vi "test_read-nmea-data2.vi"() -> ()   [LabVIEW 2019] (continued)
64,049,27,1*67\n\t\n15:12:51.40\tF9P\t$GPGSV,3,2,09,09,45,074,30,12,23,276,27,17,33,154,28,19,52,157,33,1*60\n\t\n15:12:51.42\tF9P\t$GPGSV,3,3,09,25,12,306,31,1*5E\n\t\n15:12:51.44\tF9P\t$GPGSV,3,1,09,02,55,319,,04,18,043,18,05,37,247,24,06,64,049,23,6*6C\n\t\n15:12:51.46\tF9P\t$GPGSV,3,2,09,09,45,074,27,12,23,276,,17,33,154,16,19,52,157,,6*69\n\t\n15:12:51.48\tF9P\t$GPGSV,3,3,09,25,12,306,20,6*59\n\t\n15:12:51.50\tF9P\t$GLGSV,2,1,08,69,12,031,24,70,71,039,26,71,52,205,45,72,04,209,23,1*78\n\t\n15:12:51.52\tF9P\t$GLGSV,2,2,08,77,01,326,,84,20,122,10,85,70,067,38,86,37,330,,1*72\n\t\n15:12:51.54\tF9P\t$GLGSV,2,1,08,69,12,031,17,70,71,039,,71,52,205,24,72,04,209,,3*78\n\t\n15:12:51.56\tF9P\t$GLGSV,2,2,08,77,01,326,,84,20,122,,85,70,067,21,86,37,330,,3*79\n\t\n15:12:51.58\tF9P\t$GAGSV,2,1,08,02,08,297,29,04,66,116,27,09,32,193,38,11,72,359,29,7*7B\n\t\n15:12:51.60\tF9P\t$GAGSV,2,2,08,12,40,103,33,19,26,045,19,25,09,249,,36,26,308,23,7*71\n\t\n15:12:51.62\tF9P\t$GAGSV,2,1,08,02,08,297,,04,66,116,,09,32,193,,11,72,359,,2*70\n\t\n15:12:51.64\tF9P\t$GAGSV,2,2,08,12,40,103,,19,26,045,,25,09,249,,36,26,308,,2*7D\n\t\n15:12:51.66\tF9P\t$GBGSV,1,1,04,11,49,132,31,14,87,114,28,28,,,22,33,61,220,33,1*44\n\t\n15:12:51.68\tF9P\t$GBGSV,1,1,04,10,,,33,11,49,132,,14,87,114,,33,61,220,,3*45\n\t\n15:12:51.70\tF9P\t$GNGLL,3723.54935,N,12656.96073,E,061253.00,A,A*72\n\t\n15:12:51.72\tF9P\t\t\n15:12:51.74\tF9P\t\t\n15:12:51.76\tF9P\t\t\n15:12:51.78\tF9P\t\t\n15:12:51.80\tF9P\t\t\n15:12:51.82\tF9P\t\t\n15:12:51.84\tF9P\t\t\n15:12:51.86\tF9P\t\t\n15:12:51.88\tF9P\t\t\n15:12:51.90\tF9P\t\t\n15:12:51.92\tF9P\t\t\n15:12:51.94\tF9P\t\t\n15:12:51.96\tF9P\t\t\n15:12:51.98\tF9P\t\t\n15:12:52.00\tF9P\t\t\n15:12:52.02\tF9P\t\t\n15:12:52.04\tF9P\t\t\n15:12:52.06\tF9P\t\t\n15:12:52.08\tF9P\t\t\n15:12:52.10\tF9P\t\t\n15:12:52.12\tF9P\t\t\n15:12:52.14\tF9P\t\t\n15:12:52.16\tF9P\t\t\n15:12:52.18\tF9P\t\t\n15:12:52.20\tF9P\t\t\n15:12:52.22\tF9P\t\t\n15:12:52.24\tF9P\t$GNRMC,061254.00,A,3723.54957,N,12656.96127,E,1.207,58.71,250720,,,A,V*31\n\t\n15:12:52.26\tF9P\t$GNVTG,58.71,T,,M,1.207,N,2.236,K,A*19\n\t\n15:12:52.28\tF9P\t$GNGGA,061254.00,3723.54957,N,12656.96127,E,1,12,0.83,44.6,M,18.5,M,,*76\n\t\n15:12:52.30\tF9P\t$GNGSA,A,3,06,19,05,17,09,04,02,,,,,,1.56,0.83,1.32,1*0A\n\t\n15:12:52.32\tF9P\t$GNGSA,A,3,85,70,71,84,,,,,,,,,1.56,0.83,1.32,2*0B\n\t\n15:12:52.34\tF9P\t$GNGSA,A,3,36,19,11,04,09,12,,,,,,,1.56,0.83,1.32,3*09\n\t\n15:12:52.36\tF9P\t$GNGSA,A,3,14,11,33,,,,,,,,,,1.56,0.83,1.32,4*08\n\t\n15:12:52.38\tF9P\t$GPGSV,3,1,09,02,55,319,22,04,18,043,26,05,37,247,38,06,64,049,31,1*68\n\t\n15:12:52.40\tF9P\t$GPGSV,3,2,09,09,45,074,25,12,23,276,,17,33,154,28,19,52,157,35,1*67\n\t\n15:12:52.42\tF9P\t$GPGSV,3,3,09,25,12,306,24,1*5A\n\t\n15:12:52.44\tF9P\t$GPGSV,3,1,09,02,55,319,,04,18,043,18,05,37,247,23,06,64,049,25,6*6D\n\t\n15:12:52.46\tF9P\t$GPGSV,3,2,09,09,45,074,26,12,23,276,24,17,33,154,16,19,52,157,,6*6E\n\t\n15:12:52.48\tF9P\t$GPGSV,3,3,09,25,12,306,,6*5B\n\t\n15:12:52.50\tF9P\t$GLGSV,2,1,08,69,12,031,24,70,71,039,25,71,52,205,40,72,04,209,24,1*79\n\t\n15:12:52.52\tF9P\t$GLGSV,2,2,08,77,01,326,,84,20,122,14,85,70,067,31,86,37,330,,1*7F\n\t\n15:12:52.54\tF9P\t$GLGSV,2,1,08,69,12,031,16,70,71,039,,71,52,205,25,72,04,209,,3*78\n\t\n15:12:52.56\tF9P\t$GLGSV,2,2,08,77,01,326,,84,20,122,,85,70,067,22,86,37,330,,3*7A\n\t\n15:12:52.58\tF9P\t$GAGSV,2,1,08,02,08,297,26,04,66,116,32,09,32,193,39,11,72,359,33,7*7A\n\t\n15:12:52.60\tF9P\t$GAGSV,2,2,08,12,40,103,29,19,26,045,18,25,09,249,,36,26,308,22,7*7A\n\t\n15:12:52.62\tF9P\t$GAGSV,2,1,08,02,08,297,,04,66,116,,09,32,193,,11,72,359,,2*70\n\t\n15:12:52.64\tF9P\t$GAGSV,2,2,08,12,40,103,,19,26,045,,25,09,249,,36,26,308,,2*7D\n\t\n15:12:52.66\tF9P\t$GBGSV,1,1,04,11,49,132,31,14,87,114,29,28,,,25,33,61,220,30,1*41\n\t\n15:12:52.68\tF9P\t$GBGSV,1,1,04,10,,,32,11,49,132,,14,87,114,28,33,61,220,,3*4E\n\t\n15:12:52.70\tF9P\t$GNGLL,3723.54957,N,12656.96127,E,061254.00,A,A*71\n\t\n15:12:52.72\tF9P\t\t\n15:12:52.74\tF9P\t\t\n15:12:52.76\tF9P\t\t\n15:12:52.78\tF9P\t\t\n15:12:52.80\tF9P\t\t\n15:12:52.82\tF9P\t\t\n15:12:52.84\tF9P\t\t\n15:12:52.86\tF9P\t\t\n15:12:52.88\tF9P\t\t\n15:12:52.90\tF9P\t\t\n15:12:52.92\tF9P\t\t\n15:12:52.94\tF9P\t\t\n15:12:52.96\tF9P\t\t\n15:12:52.98\tF9P\t\t\n15:12:53.01\tF9P\t\t\n15:12:53.03\tF9P\t\t\n15:12:53.05\tF9P\t\t\n15:12:53.07\tF9P\t\t\n15:12:53.09\tF9P\t\t\n15:12:53.11\tF9P\t\t\n15:12:53.13\tF9P\t\t\n15:12:53.15\tF9P\t\t\n15:12:53.17\tF9P\t\t\n15:12:53.19\tF9P\t\t\n15:12:53.21\tF9P\t\t\n15:12:53.23\tF9P\t$GNRMC,061255.00,A,3723.54950,N,12656.96154,E,1.143,,250720,,,A,V*15\n\t\n15:12:53.25\tF9P\t$GNVTG,,T,,M,1.143,N,2.116,K,A*3E\n\t\n15:12:53.27\tF9P\t$GNGGA,061255.00,3723.54950,N,12656.96154,E,1,12,0.85,43.7,M,18.5,M,,*74\n\t\n15:12:53.29\tF9P\t$GNGSA,A,3,12,06,19,05,17,09,04,02,,,,,1.68,0.85,1.45,1*02\n\t\n15:12:53.31\tF9P\t$GNGSA,A,3,85,70,71,84,,,,,,,,,1.68,0.85,1.45,2*00\n\t\n15:12:53.33\tF9P\t$GNGSA,A,3,36,19,11,04,09,12,,,,,,,1.68,0.85,1.45,3*02\n\t\n15:12:53.35\tF9P\t$GNGSA,A,3,14,11,33,,,,,,,,,,1.68,0.85,1.45,4*03\n\t\n15:12:53.37\tF9P\t$GPGSV,3,1,09,02,55,319,22,04,18,043,25,05,37,247,30,06,64,049,27,1*64\n\t\n15:12:53.39\tF9P\t$GPGSV,3,2,09,09,45,074,27,12,23,276,36,17,33,154,28,19,52,157,30,1*65\n\t\n15:12:53.41\tF9P\t$GPGSV,3,3,09,25,12,306,24,1*5A\n\t\n15:12:53.43\tF9P\t$GPGSV,3,1,09,02,55,319,,04,18,043,18,05,37,247,21,06,64,049,24,6*6E\n\t\n15:12:53.45\tF9P\t$GPGSV,3,2,09,09,45,074,25,12,23,276,22,17,33,154,16,19,52,157,,6*6B\n\t\n15:12:53.47\tF9P\t$GPGSV,3,3,09,25,12,306,,6*5B\n\t\n15:12:53.49\tF9P\t$GLGSV,2,1,08,69,12,031,25,70,71,039,31,71,52,205,40,72,04,209,24,1*7D\n\t\n15:12:53.51\tF9P\t$GLGSV,2,2,08,77,01,326,,84,20,122,10,85,70,067,37,86,37,330,,1*7D\n\t\n15:12:53.53\tF9P\t$GLGSV,2,1,08,69,12,031,16,70,71,039,,71,52,205,25,72,04,209,,3*78\n\t\n15:12:53.55\tF9P\t$GLGSV,2,2,08,77,01,326,,84,20,122,,85,70,067,21,86,37,330,,3*79\n\t\n15:12:53.57\tF9P\t$GAGSV,2,1,08,02,08,297,22,04,66,116,31,09,32,193,31,11,72,359,23,7*74\n\t\n15:12:53.59\tF9P\t$GAGSV,2,2,08,12,40,103,28,19,26,045,18,25,09,249,,36,26,308,21,7*78\n\t\n15:12:53.61\tF9P\t$GAGSV,2,1,08,02,08,297,,04,66,116,,09,32,193,33,11,72,359,,2*70\n\t\n15:12:53.63\tF9P\t$GAGSV,2,2,08,12,40,103,,19,26,045,,25,09,249,,36,26,308,,2*7D\n\t\n15:12:53.65\tF9P\t$GBGSV,1,1,04,11,49,132,28,14,87,114,28,28,,,24,33,61,220,31,1*48\n\t\n15:12:53.67\tF9P\t$GBGSV,1,1,04,10,,,28,11,49,132,28,14,87,114,26,33,61,220,,3*41\n\t\n15:12:53.69\tF9P\t$GNGLL,3723.54950,N,12656.96154,E,061255.00,A,A*73\n\t\n15:12:53.71\tF9P\t\t\n15:12:53.73\tF9P\t\t\n15:12:53.75\tF9P\t\t\n15:12:53.77\tF9P\t\t\n15:12:53.79\tF9P\t\t\n15:12:53.81\tF9P\t\t\n15:12:53.83\tF9P\t\t\n15:12:53.85\tF9P\t\t\n15:12:53.87\tF9P\t\t\n15:12:53.89\tF9P\t\t\n15:12:53.91\tF9P\t\t\n15:12:53.93\tF9P\t\t\n15:12:53.95\tF9P\t\t\n15:12:53.97\tF9P\t\t\n15:12:53.99\tF9P\t\t\n15:12:54.01\tF9P\t\t\n15:12:54.03\tF9P\t\t\n15:12:54.05\tF9P\t\t\n15:12:54.07\tF9P\t\t\n15:12:54.09\tF9P\t\t\n15:12:54.11\tF9P\t\t\n15:12:54.13\tF9P\t\t\n15:12:54.15\tF9P\t\t\n15:12:54.17\tF9P\t\t\n15:12:54.19\tF9P\t\t\n15:12:54.21\tF9P\t\t\n15:12:54.23\tF9P\t$GNRMC,061256.00,A,3723.54971,N,12656.96183,E,1.192,,250720,,,A,V*13\n\t\n15:12:54.25\tF9P\t$GNVTG,,T,,M,1.192,N,2.208,K,A*3E\n\t\n15:12:54.27\tF9P\t$GNGGA,061256.00,3723.54971,N,12656.96183,E,1,12,0.94,42.7,M,18.5,M,,*7F\n\t\n15:12:54.29\tF9P\t$GNGSA,A,3,12,06,19,05,17,09,04,02,,,,,1.64,0.94,1.34,1*08\n\t\n15:12:54.31\tF9P\t$GNGSA,A,3,85,70,71,84,,,,,,,,,1.64,0.94,1.34,2*0A\n\t\n15:12:54.33\tF9P\t$GNGSA,A,3,36,19,11,04,09,12,,,,,,,1.64,0.94,1.34,3*08\n\t\n15:12:54.35\tF9P\t$GNGSA,A,3,14,11,33,,,,,,,,,,1.64,0.94,1.34,4*09\n\t\n15:12:54.37\tF9P\t$GPGSV,3,1,09,02,55,319,22,04,18,043,26,05,37,247,33,06,64,049,27,1*64\n\t\n15:12:54.39\tF9P\t$GPGSV,3,2,09,09,45,074,31,12,23,276,,17,33,154,32,19,52,157,31,1*6D\n\t\n15:12:54.41\tF9P\t$GPGSV,3,3,09,25,12,306,24,1*5A\n\t\n15:12:54.43\tF9P\t$GPGSV,3,1,09,02,55,319,,04,18,043,17,05,37,247,19,06,64,049,23,6*6D\n\t\n15:12:54.45\tF9P\t$GPGSV,3,2,09,09,45,074,25,12,23,276,23,17,33,154,17,19,52,157,,6*6B\n\t\n15:12:54.47\tF9P\t$GPGSV,3,3,09,25,12,306,,6*5B\n\t\n15:12:54.49\tF9P\t$GLGSV,2,1,08,69,12,031,24,70,71,039,26,71,52,205,37,72,04,209,24,1*7A\n\t\n15:12:54.51\tF9P\t$GLGSV,2,2,08,77,01,326,,84,20,122,11,85,70,067,33,86,37,330,,1*78\n\t\n15:12:54.53\tF9P\t$GLGSV,2,1,08,69,12,031,17,70,71,039,,71,52,205,24,72,04,209,,3*78\n\t\n15:12:54.55\tF9P\t$GLGSV,2,2,08,77,01,326,,84,20,122,,85,70,067,21,86,37,330,,3*79\n\t\n15:12:54.57\tF9P\t$GAGSV,2,1,08,02,08,297,18,04,66,116,30,09,32,193,38,11,72,359,30,7*77\n\t\n15:12:54.59\tF9P\t$GAGSV,2,2,08,12,40,103,29,19,26,045,18,25,09,249,,36,26,308,19,7*72\n\t\n15:12:54.61\tF9P\t$GAGSV,2,1,08,02,08,297,,04,66,116,,09,32,193,29,11,72,359,,2*7B\n\t\n15:12:54.63\tF9P\t$GAGSV,2,2,08,12,40,103,,19,26,045,,25,09,249,,36,26,308,,2*7D\n\t\n15:12:54.65\tF9P\t$GBGSV,1,1,04,11,49,132,29,14,87,114,26,28,,,22,33,61,220,37,1*47\n\t\n15:12:54.67\tF9P\t$GBGSV,1,1,04,10,,,27,11,49,132,27,14,87,114,35,33,61,220,,3*43\n\t\n15:12:54.69\tF9P\t$GNGLL,3723.54971,N,12656.96183,E,061256.00,A,A*79\n\t\n15:12:54.71\tF9P\t\t\n15:12:54.73\tF9P\t\t\n15:12:54.75\tF9P\t\t\n15:12:54.77\tF9P\t\t\n15:12:54.79\tF9P\t\t\n15:12:54.81\tF9P\t\t\n15:12:54.83\tF9P\t\t\n15:12:54.85\tF9P\t\t\n15:12:54.87\tF9P\t\t\n15:12:54.89\tF9P\t\t\n15:12:54.91\tF9P\t\t\n15:12:54.93\tF9P\t\t\n15:12:54.95\tF9P\t\t\n15:12:54.97\tF9P\t\t\n15:12:54.99\tF9P\t\t\n15:12:55.01\tF9P\t\t\n15:12:55.03\tF9P\t\t\n15:12:55.05\tF9P\t\t\n15:12:55.07\tF9P\t\t\n15:12:55.09\tF9P\t\t\n15:12:55.11\tF9P\t\t\n15:12:55.13\tF9P\t\t\n15:12:55.15\tF9P\t\t\n15:12:55.17\tF9P\t\t\n15:12:55.19\tF9P\t\t\n15:12:55.21\tF9P\t\t\n15:12:55.23\tF9P\t$GNRMC,061257.00,A,3723.55023,N,12656.96251,E,2.718,53.97,250720,,,A,V*30\n\t\n15:12:55.25\tF9P\t$GNVTG,53.97,T,,M,2.718,N,5.033,K,A*12\n\t\n15:12:55.27\tF9P\t$GNGGA,061257.00,3723.55023,N,12656.96251,E,1,12,0.93,42.5,M,18.5,M,,*78\n\t\n15:12:55.29\tF9P\t$GNGSA,A,3,12,06,19,05,17,09,04,02,,,,,1.63,0.93,1.34,1*08\n\t\n15:12:55.31\tF9P\t$GNGSA,A,3,85,70,71,84,,,,,,,,,1.63,0.93,1.34,2*0A\n\t\n15:12:55.33\tF9P\t$GNGSA,A,3,36,19,11,04,09,12,,,,,,,1.63,0.93,1.34,3*08\n\t\n15:12:55.35\tF9P\t$GNGSA,A,3,14,11,33,,,,,,,,,,1.63,0.93,1.34,4*09\n\t\n15:12:55.37\tF9P\t$GPGSV,3,1,09,02,55,319,22,04,18,043,27,05,37,247,29,06,64,049,26,1*6F\n\t\n15:12:55.39\tF9P\t$GPGSV,3,2,09,09,45,074,31,12,23,276,30,17,33,154,32,19,52,157,37,1*68\n\t\n15:12:55.41\tF9P\t$GPGSV,3,3,09,25,12,306,24,1*5A\n\t\n15:12:55.43\tF9P\t$GPGSV,3,1,09,02,55,319,,04,18,043,19,05,37,247,19,06,64,049,23,6*63\n\t\n15:12:55.45\tF9P\t$GPGSV,3,2,09,09,45,074,26,12,23,276,,17,33,154,17,19,52,157,,6*69\n\t\n15:12:55.47\tF9P\t$GPGSV,3,3,09,25,12,306,,6*5B\n\t\n15:12:55.49\tF9P\t$GLGSV,2,1,08,69,12,031,24,70,71,039,27,71,52,205,41,72,04,209,23,1*7D\n\t\n15:12:55.51\tF9P\t$GLGSV,2,2,08,77,01,326,,84,20,122,13,85,70,067,39,86,37,330,,1*70\n\t\n15:12:55.53\tF9P\t$GLGSV,2,1,08,69,12,031,17,70,71,039,,71,52,205,24,72,04,209,,3*78\n\t\n15:12:55.55\tF9P\t$GLGSV,2,2,08,77,01,326,,84,20,122,22,85,70,067,21,86,37,330,,3*79\n\t\n15:12:55.57\tF9P\t$GAGSV,2,1,08,02,08,297,19,04,66,116,28,09,32,193,32,11,72,359,30,7*75\n\t\n15:12:55.59\tF9P\t$GAGSV,2,2,08,12,40,103,30,19,26,045,19,25,09,249,,36,26,308,18,7*7A\n\t\n15:12:55.61\tF9P\t$GAGSV,2,1,08,02,08,297,,04,66,116,,09,32,193,34,11,72,359,,2*77\n\t\n15:12:55.63\tF9P\t$GAGSV,2,2,08,12,40,103,,19,26,045,,25,09,249,,36,26,308,,2*7D\n\t\n15:12:55.65\tF9P\t$GBGSV,1,1,04,11,49,132,36,14,87,114,28,28,,,21,33,61,220,36,1*45\n\t\n15:12:55.67\tF9P\t$GBGSV,1,1,03,11,49,132,29,14,87,114,,33,61,220,,3*48\n\t\n15:12:55.69\tF9P\t$GNGLL,3723.55023,N,12656.96251,E,061257.00,A,A*7B\n\t\n15:12:55.71\tF9P\t\t\n15:12:55.73\tF9P\t\t\n15:12:55.75\tF9P\t\t\n15:12:55.77\tF9P\t\t\n15:12:55.79\tF9P\t\t\n15:12:55.81\tF9P\t\t\n15:12:55.83\tF9P\t\t\n15:12:55.85\tF9P\t\t\n15:12:55.87\tF9P\t\t\n15:12:55.89\tF9P\t\t\n15:12:55.91\tF9P\t\t\n15:12:55.93\tF9P\t\t\n15:12:55.95\tF9P\t\t\n15:12:55.97\tF9P\t\t\n15:12:55.99\tF9P\t\t\n15:12:56.01\tF9P\t\t\n15:12:56.03\tF9P\t\t\n15:12:56.05\tF9P\t\t\n15:12:56.07\tF9P\t\t\n15:12:56.09\tF9P\t\t\n15:12:56.11\tF9P\t\t\n15:12:56.13\tF9P\t\t\n15:12:56.15\tF9P\t\t\n15:12:56.17\tF9P\t\t\n15:12:56.19\tF9P\t\t\n15:12:56.21\tF9P\t\t\n15:12:56.23\tF9P\t$GNRMC,061258.00,A,3723.55052,N,12656.96301,E,1.338,,250720,,,A,V*1E\n\t\n15:12:56.25\tF9P\t$GNVTG,,T,,M,1.338,N,2.478,K,A*3D\n\t\n15:12:56.27\tF9P\t$GNGGA,061258.00,3723.55052,N,12656.96301,E,1,12,0.93,43.2,M,18.5,M,,*73\n\t\n15:12:56.29\tF9P\t$GNGSA,A,3,06,19,05,17,09,04,02,,,,,,1.63,0.93,1.34,1*0B\n\t\n15:12:56.31\tF9P\t$GNGSA,A,3,85,70,71,84,,,,,,,,,1.63,0.93,1.34,2*0A\n\t\n15:12:56.33\tF9P\t$GNGSA,A,3,36,19,11,04,09,12,,,,,,,1.63,0.93,1.34,3*08\n\t\n15:12:56.35\tF9P\t$GNGSA,A,3,14,11,33,,,,,,,,,,1.63,0.93,1.34,4*09\n\t\n15:12:56.37\tF9P\t$GPGSV,3,1,09,02,55,319,22,04,18,043,26,05,37,247,29,06,64,049,32,1*6B\n\t\n15:12:56.39\tF9P\t$GPGSV,3,2,09,09,45,074,30,12,23,276,,17,33,154,31,19,52,157,30,1*6E\n\t\n15:12:56.41\tF9P\t$GPGSV,3,3,09,25,12,306,22,1*5C\n\t\n15:12:56.43\tF9P\t$GPGSV,3,1,09,02,55,319,,04,18,043,20,05,37,247,19,06,64,049,24,6*6E\n\t\n15:12:56.45\tF9P\t$GPGSV,3,2,09,09,45,074,26,12,23,276,26,17,33,154,18,19,52,157,,6*62\n\t\n15:12:56.47\tF9P\t$GPGSV,3,3,09,25,12,306,,6*5B\n\t\n15:12:56.49\tF9P\t$GLGSV,2,1,08,69,11,031,23,70,71,039,31,71,52,205,36,72,04,209,22,1*7F\n\t\n15:12:56.51\tF9P\t$GLGSV,2,2,08,77,01,326,,84,20,122,17,85,70,067,39,86,37,330,,1*74\n\t\n15:12:56.53\tF9P\t$GLGSV,2,1,08,69,11,031,17,70,71,039,,71,52,205,25,72,04,209,,3*7A\n\t\n15:12:56.55\tF9P\t$GLGSV,2,2,08,77,01,326,,84,20,122,21,85,70,067,22,86,37,330,,3*79\n\t\n15:12:56.57\tF9P\t$GAGSV,2,1,08,02,08,297,17,04,66,116,27,09,32,193,35,11,72,359,33,7*70\n\t\n15:12:56.59\tF9P\t$GAGSV,2,2,08,12,40,103,29,19,26,045,21,25,09,249,,36,26,308,18,7*79\n\t\n15:12:56.61\tF9P\t$GAGSV,2,1,08,02,08,297,,04,66,116,,09,32,193,28,11,72,359,,2*7A\n\t\n15:12:56.63\tF9P\t$GAGSV,2,2,08,12,40,103,,19,26,045,,25,09,249,,36,26,308,,2*7D\n\t\n15:12:56.65\tF9P\t$GBGSV,1,1,04,11,49,132,30,14,87,114,31,28,,,19,33,61,220,30,1*46\n\t\n15:12:56.67\tF9P\t$GBGSV,1,1,03,11,49,132,28,14,87,114,,33,61,220,,3*49\n\t\n15:12:56.69\tF9P\t$GNGLL,3723.55052,N,12656.96301,E,061258.00,A,A*76\n\t\n15:12:56.71\tF9P\t\t\n15:12:56.73\tF9P\t\t\n15:12:56.75\tF9P\t\t\n15:12:56.77\tF9P\t\t\n15:12:56.79\tF9P\t\t\n15:12:56.81\tF9P\t\t\n15:12:56.83\tF9P\t\t\n15:12:56.85\tF9P\t\t\n15:12:56.87\tF9P\t\t\n15:12:56.89\tF9P\t\t\n15:12:56.91\tF9P\t\t\n15:12:56.93\tF9P\t\t\n15:12:56.95\tF9P\t\t\n15:12:56.97\tF9P\t\t\n15:12:56.99\tF9P\t\t\n15:12:57.01\tF9P\t\t\n15:12:57.03\tF9P\t\t\n15:12:57.05\tF9P\t\t\n15:12:57.07\tF9P\t\t\n15:12:57.09\tF9P\t\t\n15:12:57.11\tF9P\t\t\n15:12:57.13\tF9P\t\t\n15:12:57.15\tF9P\t\t\n15:12:57.17\tF9P\t\t\n15:12:57.19\tF9P\t\t\n15:12:57.21\tF9P\t\t\n15:12:57.23\tF9P\t$GNRMC,061259.00,A,3723.55105,N,12656.96385,E,2.117,53.68,250720,,,A,V*3A\n\t\n15:12:57.25\tF9P\t$GNVTG,53.68,T,,M,2.117,N,3.920,K,A*16\n\t\n15:12:57.27\tF9P\t$GNGGA,061259.00,3723.55105,N,12656.96385,E,1,12,0.94,41.7,M,18.5,M,,*7D\n\t\n15:12:57.29\tF9P\t$GNGSA,A,3,06,19,05,17,09,04,02,,,,,,1.64,0.94,1.34,1*0B\n\t\n15:12:57.31\tF9P\t$GNGSA,A,3,85,70,71,84,,,,,,,,,1.64,0.94,1.34,2*0A\n\t\n15:12:57.33\tF9P\t$GNGSA,A,3,36,19,11,04,09,12,,,,,,,1.64,0.94,1.34,3*08\n\t\n15:12:57.35\tF9P\t$GNGSA,A,3,14,11,33,,,,,,,,,,1.64,0.94,1.34,4*09\n\t\n15:12:57.37\tF9P\t$GPGSV,3,1,09,02,55,319,23,04,18,043,25,05,37,247,31,06,64,049,30,1*62\n\t\n15:12:57.39\tF9P\t$GPGSV,3,2,09,09,45,074,34,12,23,276,26,17,33,154,33,19,52,157,30,1*6C\n\t\n15:12:57.41\tF9P\t$GPGSV,3,3,09,25,12,306,22,1*5C\n\t\n15:12:57.43\tF9P\t$GPGSV,3,1,09,02,55,319,,04,18,043,19,05,37,247,20,06,64,049,22,6*68\n\t\n15:12:57.45\tF9P\t$GPGSV,3,2,09,09,45,074,30,12,23,276,23,17,33,154,20,19,52,157,,6*6B\n\t\n15:12:57.47\tF9P\t$GPGSV,3,3,09,25,12,306,,6*5B\n\t\n15:12:57.49\tF9P\t$GLGSV,2,1,08,69,11,031,30,70,70,038,30,71,52,205,42,72,04,209,22,1*7F\n\t\n15:12:57.51\tF9P\t$GLGSV,2,2,08,77,01,326,,84,20,122,14,85,70,067,31,86,37,330,,1*7F\n\t\n15:12:57.53\tF9P\t$GLGSV,2,1,08,69,11,031,16,70,70,038,,71,52,205,24,72,04,209,,3*7A\n\t\n15:12:57.55\tF9P\t$GLGSV,2,2,08,77,01,326,,84,20,122,20,85,70,067,22,86,37,330,,3*78\n\t\n15:12:57.57\tF9P\t$GAGSV,2,1,08,02,08,297,15,04,66,116,26,09,32,193,35,11,72,359,28,7*79\n\t\n15:12:57.59\tF9P\t$GAGSV,2,2,08,12,40,103,38,19,26,045,20,25,09,249,,36,26,308,18,7*78\n\t\n15:12:57.61\tF9P\t$GAGSV,2,1,08,02,08,297,,04,66,116,,09,32,193,31,11,72,359,,2*72\n\t\n15:12:57.63\tF9P\t$GAGSV,2,2,08,12,40,103,,19,26,045,,25,09,249,,36,26,308,,2*7D\n\t\n15:12:57.65\tF9P\t$GBGSV,1,1,04,11,49,132,34,14,87,114,31,28,,,18,33,61,220,32,1*41\n\t\n15:12:57.67\tF9P\t$GBGSV,1,1,03,11,49,132,,14,87,114,,33,61,220,,3*43\n\t\n15:12:57.69\tF9P\t$GNGLL,3723.55105,N,12656.96385,E,061259.00,A,A*78\n\t\n15:12:57.71\tF9P\t\t\n15:12:57.73\tF9P\t\t\n15:12:57.75\tF9P\t\t\n15:12:57.77\tF9P\t\t\n15:12:57.79\tF9P\t\t\n15:12:57.81\tF9P\t\t\n15:12:57.83\tF9P\t\t\n15:12:57.85\tF9P\t\t\n15:12:57.87\tF9P\t\t\n15:12:57.89\tF9P\t\t\n15:12:57.91\tF9P\t\t\n15:12:57.93\tF9P\t\t\n15:12:57.95\tF9P\t\t\n15:12:57.97\tF9P\t\t\n15:12:57.99\tF9P\t\t\n15:12:58.01\tF9P\t\t\n15:12:58.03\tF9P\t\t\n15:12:58.05\tF9P\t\t\n15:12:58.07\tF9P\t\t\n15:12:58.09\tF9P\t\t\n15:12:58.11\tF9P\t\t\n15:12:58.13\tF9P\t\t\n15:12:58.15\tF9P\t\t\n15:12:58.17\tF9P\t\t\n15:12:58.19\tF9P\t\t\n15:12:58.21\tF9P\t\t\n15:12:58.23\tF9P\t$GNRMC,061300.00,A,3723.55141,N,12656.96468,E,2.231,58.32,250720,,,A,V*30\n\t\n15:12:58.25\tF9P\t$GNVTG,58.32,T,,M,2.231,N,4.133,K,A*18\n\t\n15:12:58.27\tF9P\t$GNGGA,061300.00,3723.55141,N,12656.96468,E,1,12,0.93,41.4,M,18.5,M,,*70\n\t\n15:12:58.29\tF9P\t$GNGSA,A,3,06,19,05,17,09,04,02,,,,,,1.63,0.93,1.34,1*0B\n\t\n15:12:58.31\tF9P\t$GNGSA,A,3,85,70,71,84,,,,,,,,,1.63,0.93,1.34,2*0A\n\t\n15:12:58.33\tF9P\t$GNGSA,A,3,36,19,11,04,09,12,,,,,,,1.63,0.93,1.34,3*08\n\t\n15:12:58.35\tF9P\t$GNGSA,A,3,14,11,33,,,,,,,,,,1.63,0.93,1.34,4*09\n\t\n15:12:58.37\tF9P\t$GPGSV,3,1,09,02,55,319,21,04,18,043,31,05,37,247,26,06,64,049,31,1*62\n\t\n15:12:58.39\tF9P\t$GPGSV,3,2,09,09,45,074,28,12,23,276,25,17,33,154,32,19,52,157,30,1*63\n\t\n15:12:58.41\tF9P\t$GPGSV,3,3,09,25,12,306,22,1*5C\n\t\n15:12:58.43\tF9P\t$GPGSV,3,1,09,02,55,319,,04,18,043,20,05,37,247,23,06,64,049,23,6*60\n\t\n15:12:58.45\tF9P\t$GPGSV,3,2,09,09,45,074,29,12,23,276,19,17,33,154,20,19,52,157,,6*6A\n\t\n15:12:58.47\tF9P\t$GPGSV,3,3,09,25,12,306,,6*5B\n\t\n15:12:58.49\tF9P\t$GLGSV,2,1,08,69,11,031,23,70,70,038,28,71,53,206,40,72,04,209,21,1*77\n\t\n15:12:58.51\tF9P\t$GLGSV,2,2,08,77,01,326,,84,20,122,15,85,70,067,26,86,37,330,,1*78\n\t\n15:12:58.53\tF9P\t$GLGSV,2,1,08,69,11,031,15,70,70,038,,71,53,206,25,72,04,209,,3*7A\n\t\n15:12:58.55\tF9P\t$GLGSV,2,2,08,77,01,326,,84,20,122,19,85,70,067,22,86,37,330,,3*72\n\t\n15:12:58.58\tF9P\t$GAGSV,2,1,08,02,08,297,12,04,66,116,32,09,32,193,34,11,72,359,28,7*7A\n\t\n15:12:58.60\tF9P\t$GAGSV,2,2,08,12,40,103,32,19,26,045,22,25,09,249,,36,26,308,17,7*7F\n\t\n15:12:58.62\tF9P\t$GAGSV,2,1,08,02,08,297,,04,66,116,,09,32,193,31,11,72,359,,2*72\n\t\n15:12:58.64\tF9P\t$GAGSV,2,2,08,12,40,103,,19,26,045,,25,09,249,,36,26,308,,2*7D\n\t\n15:12:58.66\tF9P\t$GBGSV,1,1,04,11,49,132,30,14,87,114,28,28,,,19,33,61,220,28,1*47\n\t\n15:12:58.68\tF9P\t$GBGSV,1,1,03,11,49,132,,14,87,114,,33,61,220,,3*43\n\t\n15:12:58.70\tF9P\t$GNGLL,3723.55141,N,12656.96468,E,061300.00,A,A*71\n\t\n15:12:58.72\tF9P\t\t\n15:12:58.74\tF9P\t\t\n15:12:58.76\tF9P\t\t\n15:12:58.78\tF9P\t\t\n15:12:58.80\tF9P\t\t\n15:12:58.82\tF9P\t\t\n15:12:58.84\tF9P\t\t\n15:12:58.86\tF9P\t\t\n15:12:58.88\tF9P\t\t\n15:12:58.90\tF9P\t\t\n15:12:58.92\tF9P\t\t\n15:12:58.94\tF9P\t\t\n15:12:58.96\tF9P\t\t\n15:12:58.98\tF9P\t\t\n15:12:59.00\tF9P\t\t\n15:12:59.02\tF9P\t\t\n15:12:59.04\tF9P\t\t\n15:12:59.06\tF9P\t\t\n15:12:59.08\tF9P\t\t\n15:12:59.10\tF9P\t\t\n15:12:59.12\tF9P\t\t\n15:12:59.14\tF9P\t\t\n15:12:59.16\tF9P\t\t\n15:12:59.18\tF9P\t\t\n15:12:59.20\tF9P\t\t\n15:12:59.22\tF9P\t\t\n15:12:59.24\tF9P\t$GNRMC,061301.00,A,3723.55169,N,12656.96549,E,2.140
